vi "getScript.vi"(8 "error in (no error)":errorcluster, 11 "tBSONJavaScript in":refnum<class "tBSONJavaScript.lvclass">) -> (0 "error out":errorcluster, 2 "Script":string, 3 "tBSONJavaScript out":refnum<class "tBSONJavaScript.lvclass">)   [LabVIEW 2013, in "BSON.lvlib" / "tBSONJavaScript.lvclass"]
uses:
  tBSONJavaScript.lvclass
  tBSONJavaScript.lvclass/tBSONJavaScript.ctl
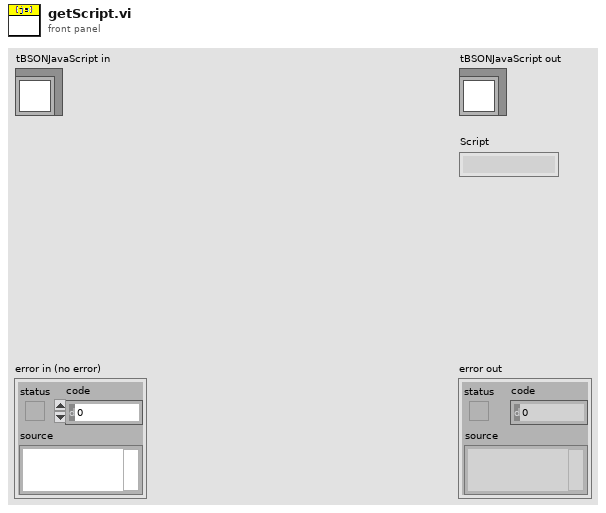
[diagram p1: front panel]
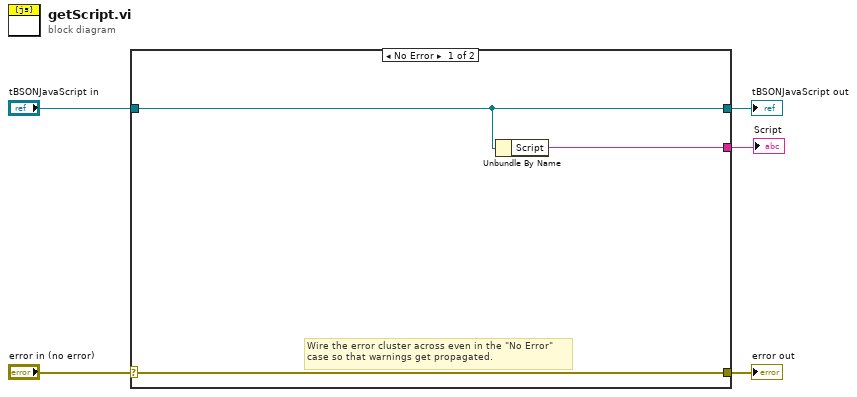
[diagram p0: block diagram]
diagram:
  n1 = case shown="No Error" "error in (no error)" {
    selector: "error in (no error)" -> [w8 w10]
    tunnel: [w8 w10] -> w4
    tunnel: [w7 w9] -> w2
    tunnel: "tBSONJavaScript in" -> [w7 w9]
    tunnel: [w6 _] -> w1
    frame No Error {
      # "Wire the error cluster across even in the \"No Error\"\ncase so that warnings get propagated."
      n2 = Unbundle By Name(w7) -> ("Script"=w6:string)
    }
    frame Error {
    }
  }
  "error out" <- w4
  "tBSONJavaScript out" <- w2
  "Script" <- w1
